vi "MakeFilter_v0.vi"(8 "error in (no error)":errorcluster, 11 "Image":T1=refnum) -> (0 "error out":errorcluster, 3 "Image Out":T1)   [LabVIEW 2017]
uses:
  <vilib>/vision/Image Controls.llb/IMAQ Image.ctl
  <vilib>/Analysis/_algsub.llb/Vector Norm Type.ctl
  <vilib>/Analysis/_algsub.llb/Real Vector Norm.vi
  <vilib>/Analysis/NI_AALPro.lvlib
panel:
  in  "dx,dy":i8[](array[numeric])=[-6, -1]
  in  "multiplier":dbl=1.025
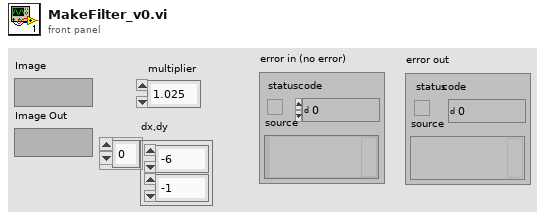
[diagram p1: front panel]
types:
  T1 = typedef "IMAQ Image.ctl" = refnum<image>
  T2 = typedef "Image Type" = u32
  T3 = typedef "NI_AALPro.lvlib/Vector Norm Type.ctl" = u16
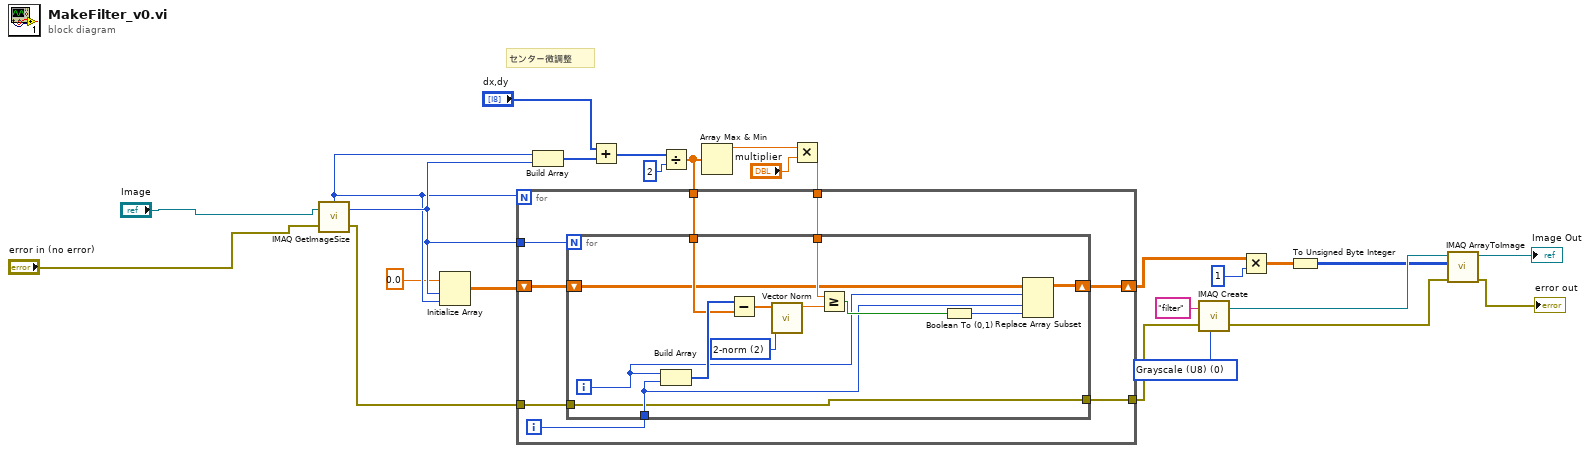
[diagram p0: block diagram]
diagram:
  w6 = T2 0 items=["Grayscale (U8)", "Grayscale (I16)", "Grayscale (SGL)", "Complex (CSG)", "RGB (U32)", "HSL (U32)", "RGB (U64)", "Grayscale (U16)"] ("Image Type")
  # "センター微調整"
  n1 = call "IMAQ GetImageSize"("Image"="Image", "error in (no error)"="error in (no error)") -> ("Y Resolution"=w22:i32, "X Resolution"=w21:i32, "error out"=w20:errorcluster)  [unwired: 2 in]
  n2 = Initialize Array(0.0, w22, w21) -> (w18:dbl[][])
  n3 = Build Array(w21, w22) -> (w26:i32[])
  n4 = Add(x="dx,dy", y=w26) -> (x+y=w2:i32[])
  n5 = Divide(x=w2, y=2) -> (x/y=w24:dbl[])
  n6 = Array Max & Min(array=w24) -> (max value=w23:dbl)  [unwired: 3 out]
  n7 = Multiply(x=w23, y="multiplier") -> (x*y=w13:dbl)
  n8 = for {
    N: w21 -> [_]
    tunnel: w22 -> [w34]
    tunnel: w24 -> [w33]
    tunnel: w13 -> [w32]
    shift-right: [w27] -> w7
    shift-left: w18 -> [w31]
    tunnel: [w29] -> w16
    tunnel: w20 -> [w30]
    i -> [w28]
    n9 = for {
      N: w34 -> [_]
      tunnel: w28 -> [w39]
      tunnel: w33 -> [w46]
      tunnel: w32 -> [w45]
      shift-right: [w40] -> w27
      shift-left: w31 -> [w41]
      tunnel: w30 -> [w38]
      tunnel: [w38] -> w29
      i -> [w37]
      w35 = T3 2 items=["1-norm"=1, "2-norm"=2, "Inf-norm"=3, "-Inf-norm"=4, "User Defined"=5] ("norm type")
      n10 = Build Array(w37, w39) -> (w47:i32[])
      n11 = Subtract(x=w47, y=w46) -> (x-y=w44:dbl[])
      n12 = call-poly <vilib>:"Vector Norm.vi"("norm type"=w35, "Input Vector"=w44) -> ("norm"=w43:dbl)  [unwired: 8 in, 1 out]
      n13 = Greater Or Equal?(x=w45, y=w43) -> (x >= y?=w42:bool)
      n14 = Boolean To (0,1)(Boolean=w42) -> (0, 1=w36:i16)
      n15 = Replace Array Subset(array=w41, new element=w36, index (row)=w37, index (col)=w39) -> (w40:dbl[][])
    }
  }
  n16 = call "IMAQ Create"("Image Name"="filter", "Image Type"=w6, "error in (no error)"=w16) -> ("New Image"=w14:T1, "error out"=w15:errorcluster)  [unwired: 2 in]
  n17 = Multiply(x=w7, y=1) -> (x*y=w5:dbl[][])
  n18 = To Unsigned Byte Integer(number=w5) -> (unsigned 8bit integer=w3:u8[][])
  n19 = call "IMAQ ArrayToImage"("error in (no error)"=w15, "Image Pixels (U8)"=w3, "Image"=w14) -> ("error out"=→"error out":errorcluster, "Image Out"=→"Image Out":T1)  [unwired: 7 in]
